vi "SPC_clear_rates.vi"(8 "Error In":errorcluster, 10 "Module no":i16 caption="Module No" min=0 max=7 step=1, 11 "DLL Path":path) -> (0 "Error Out":errorcluster, 2 "Module  No":i16, 3 "DLL Path":path)   [LabVIEW 2023]
doc: "The procedure clears all rate counters for the specified SPC module no.\nTo get correct rate values the procedure must be called once before the first call of the\nSPC_read_rates function. SPC_clear_rates starts a new rate integration cycle.\n\ninfo@becker-hickl.com"
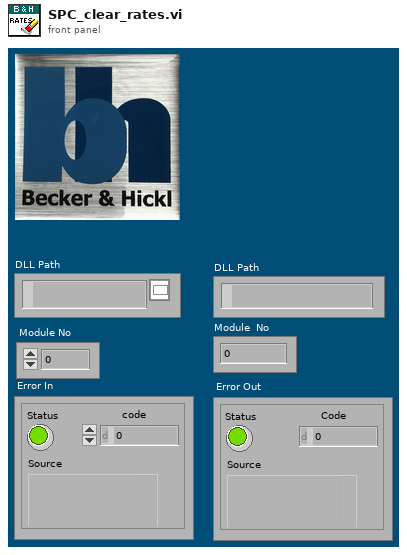
[diagram p1: front panel]
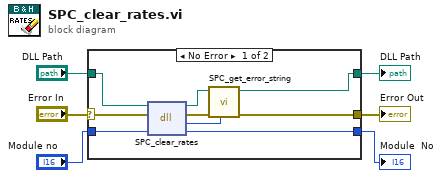
[diagram p0: block diagram]
diagram:
  n1 = case shown="No Error" "Error In" {
    selector: "Error In" -> [w13 w17]
    tunnel: [w14 w17] -> w6
    tunnel: "DLL Path" -> [w12 w18]
    tunnel: [w9 w18] -> w3
    tunnel: "Module no" -> [w8 w16]
    tunnel: [w7 w16] -> w1
    frame No Error {
      n2 = dll-call lib="D:/spcm/lib/lab_view/lv10.0/spcm32.dll" fn="SPC_clear_rates"(path in=w12, error in=w13, "mod_no"=w8) -> (path out=w10:path, error out=w15:errorcluster, "return type"=w11:i16, "mod_no"=w7:i16)  [unwired: 1 in]
      n3 = call "SPC_get_error_string.vi"("ErrorID"=w11, "Error In"=w15, "DLL Path"=w10) -> ("Error Out"=w14:errorcluster, "DLL Path"=w9:path)  [unwired: 6 in, 1 out]
    }
    frame Error {
    }
  }
  "Error Out" <- w6
  "DLL Path" <- w3
  "Module  No" <- w1
